vi "Main.vi"(11 "Args":string[](array[string])) -> (2 "Output":string, 3 "Return Status":i32)   [LabVIEW 2019, in "MicronTemplateService.lvlib"]
uses:
  MicronTemplateService.lvlib
  vi.lib/Micron/Base/Server/Service/ServiceBase.lvclass
  vi.lib/Micron/Base/Server/Service/Typedefs/MicronArgs.ctl
  Core/MicronTemplateCore.lvclass
  <vilib>/Utility/error.llb/DialogType.ctl
  <vilib>/SLL Toolkit/SLL Queued State Machine/Queue Driver/Create Queue.vi
  <vilib>/SLL Toolkit/SLL Queued State Machine/Queue Driver/Enqueue an Item to Queue.vi
  <vilib>/SLL Toolkit/SLL Queued State Machine/Queue Driver/Dequeue Queue.vi
  <vilib>/SLL Toolkit/SLL Queued State Machine/Queue Driver/Enstack an Item to Queue.vi
  Core/Methods/Add.vi
  <vilib>/SLL Toolkit/SLL Queued State Machine/Queue Driver/Enqueue N Items.vi
  <vilib>/SLL Toolkit/SLL Queued State Machine/Queue Driver/Flush Queue.vi
  <vilib>/SLL Toolkit/SLL Queued State Machine/Queue Driver/Release Queue.vi
  vi.lib/Micron/Base/Server/Message/MessageBase.lvclass
  <vilib>/SLL Toolkit/SLL Queued State Machine/SLL QSM.lvlib
  vi.lib/Micron/gRPC/Server/Service/GRPCService.lvclass
  <vilib>/SLL Toolkit/SLL String/SLL String.lvlib
panel:
  in  "Mode":enum32{"Service", "Manual"}(tab)
  in  "Connection String":string="localhost:50051"
  out "Network":string
  out "ServiceID":string
  out "Last Command":string
  out "Payload":string
  out "Last Message Timestamp":string
  in  "Command":string(combo)
  in  "Run":bool
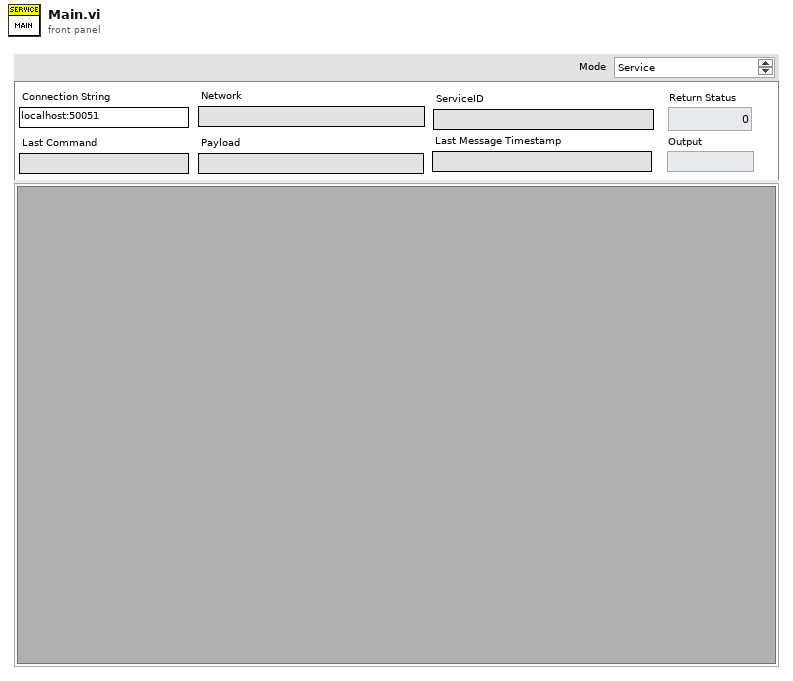
[diagram p1: front panel]
types:
  T1 = typedef "MicronServer.lvlib/ServiceBase.lvclass/MicronArgs.ctl" = cluster{"Connection":string, "Network":string, "ServiceID":string, "Port":i32, "FullyQualifiedName":string, "UI":string, "Args":string[]}
  T2 = cluster{"Flags":cluster{"Source Code?":bool}, "MicronServer":refnum<class "ServiceBase.lvclass">, "Service":T1, "UI":cluster{"Hide?":bool, "SubPanel":refnum<vi>}, "CommandMap":map{string, path}, "ManualCommandVI":refnum<vi>}
  T3 = enum32{"Invalid", "Standard", "Closed", "Hidden", "Minimized", "Maximized"}
  T4 = enum8{"Enabled", "Disabled", "Disabled and Grayed Out"}
  T5 = typedef "DialogType.ctl" = u16
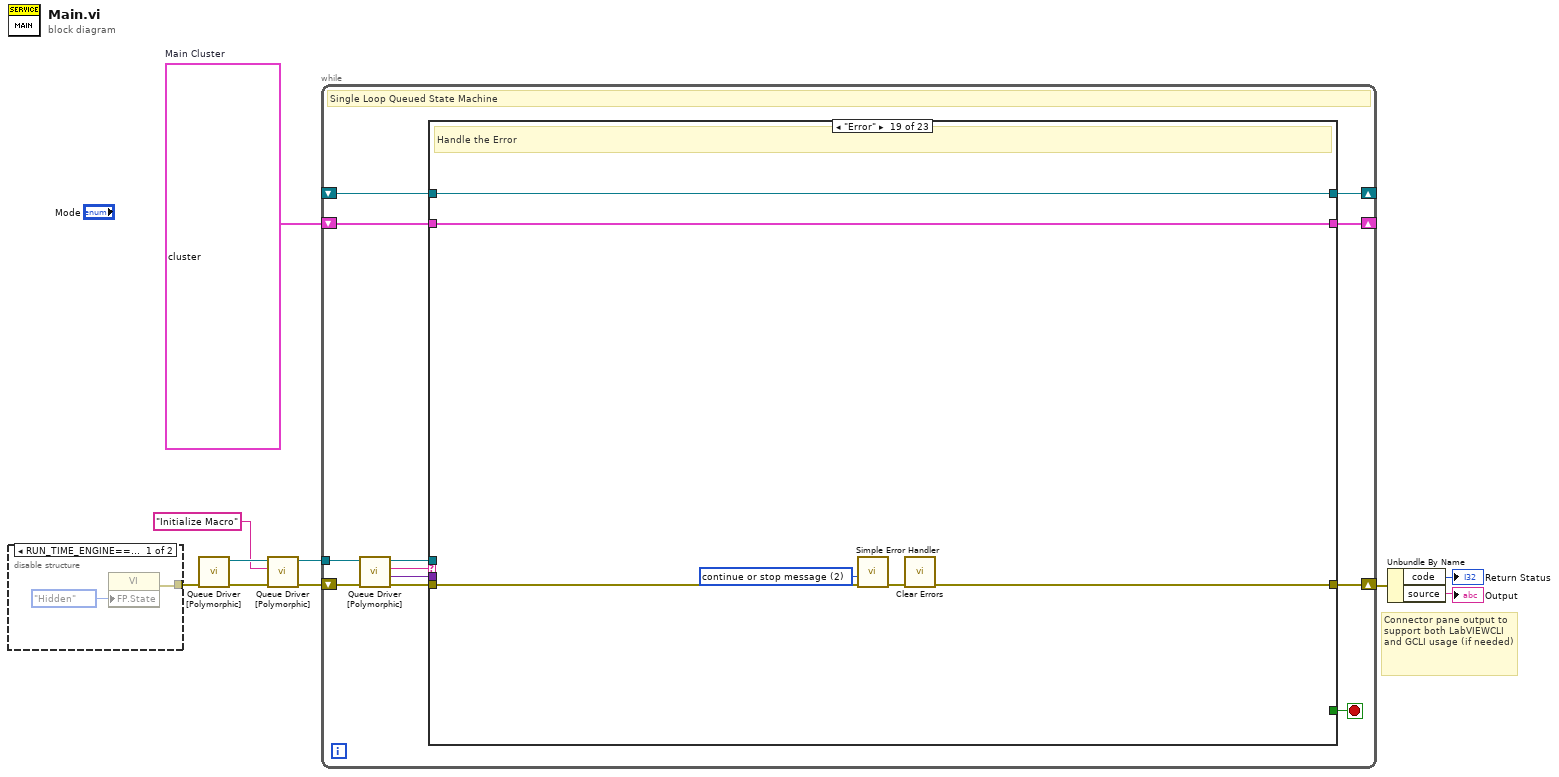
[diagram p0: block diagram]
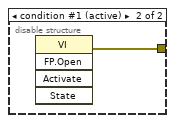
[diagram p2: hidden frame]
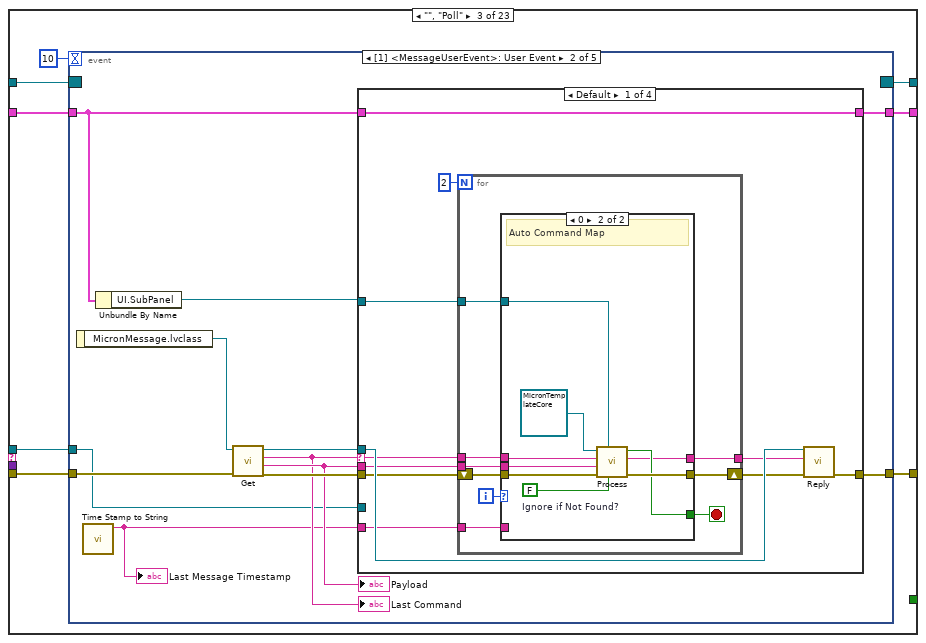
[diagram p5: hidden frame]
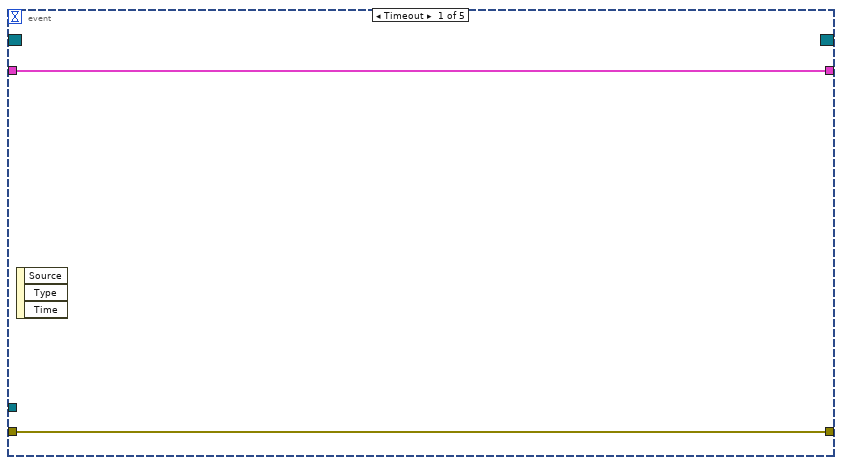
[diagram p6: hidden frame]
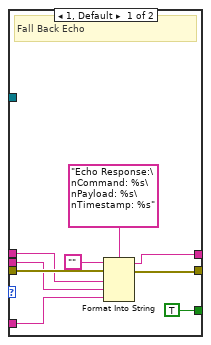
[diagram p7: hidden frame]
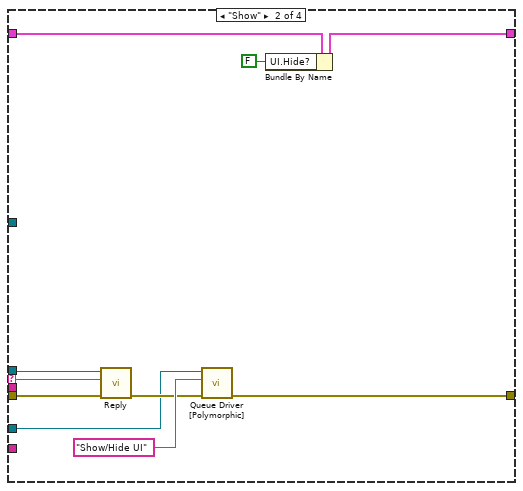
[diagram p8: hidden frame]
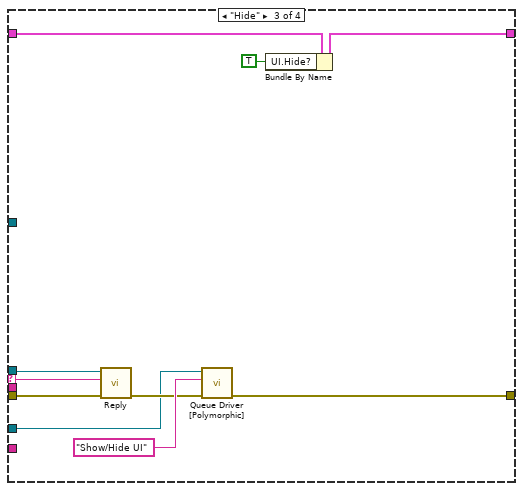
[diagram p9: hidden frame]
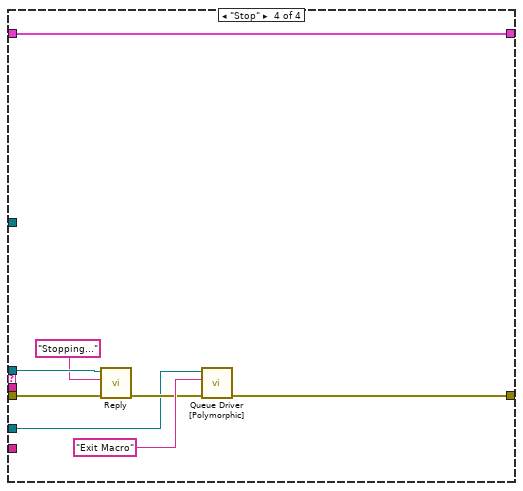
[diagram p10: hidden frame]
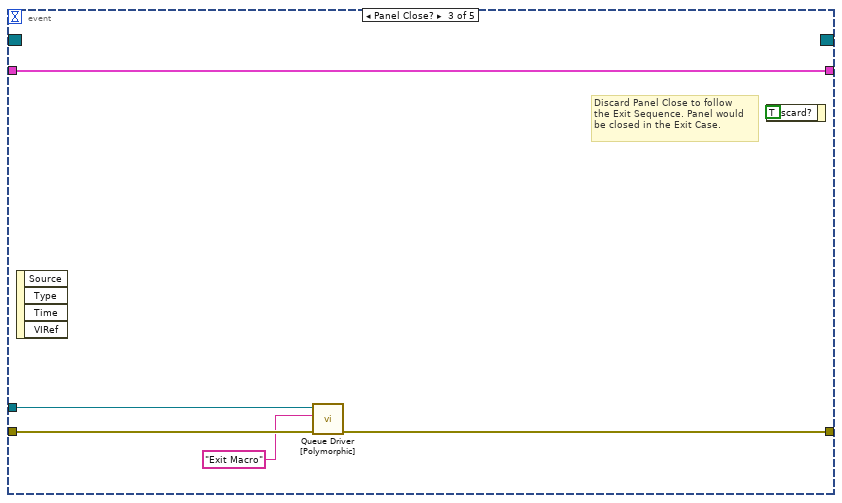
[diagram p11: hidden frame]
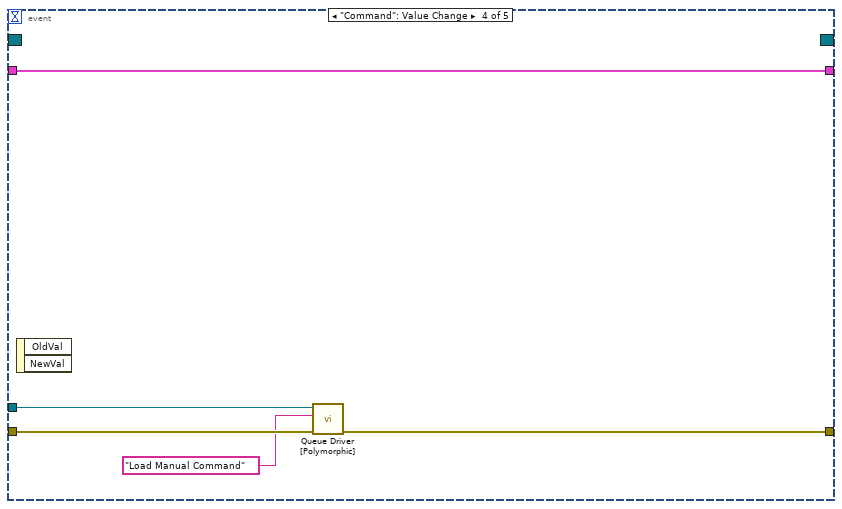
[diagram p12: hidden frame]
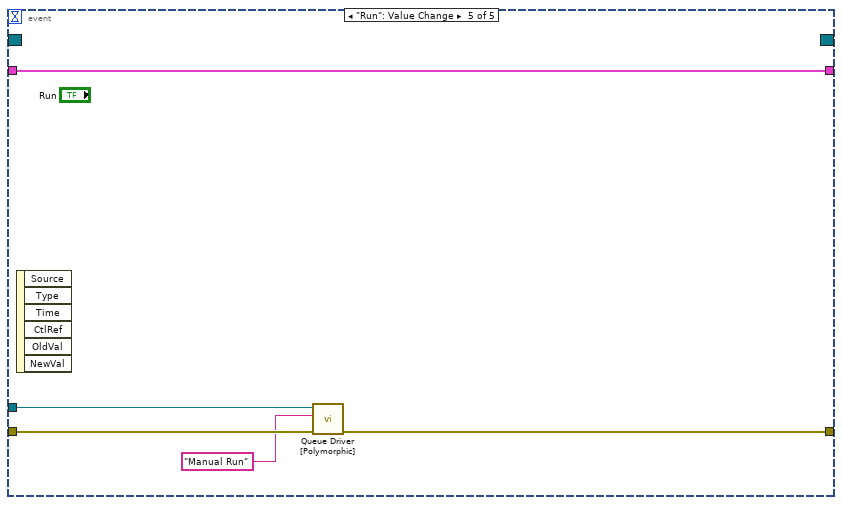
[diagram p13: hidden frame]
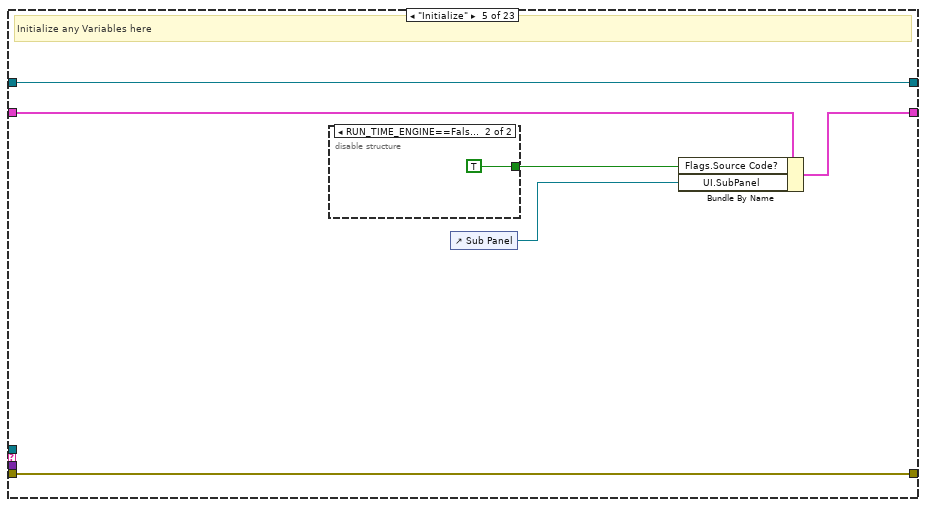
[diagram p15: hidden frame]
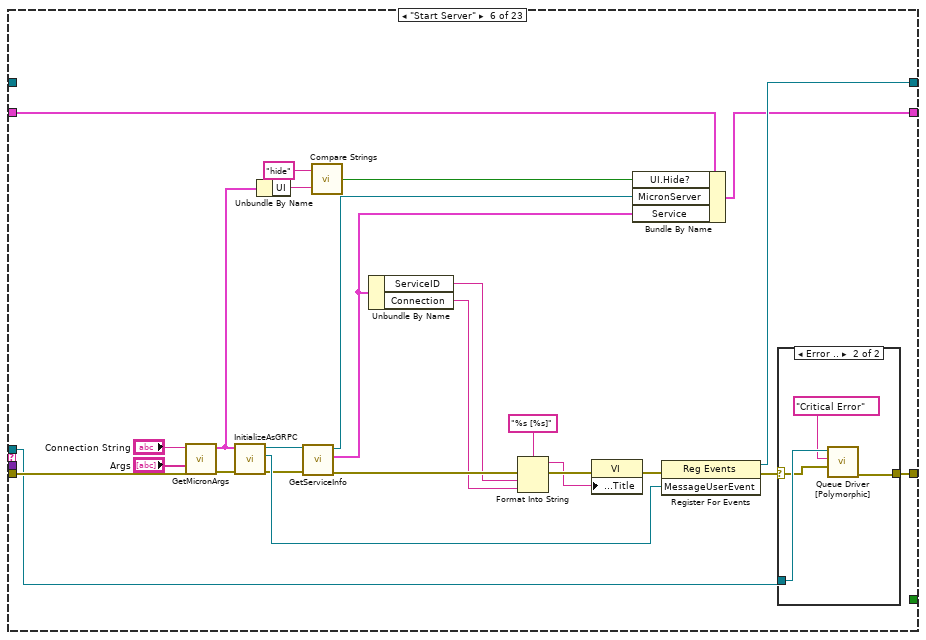
[diagram p17: hidden frame]
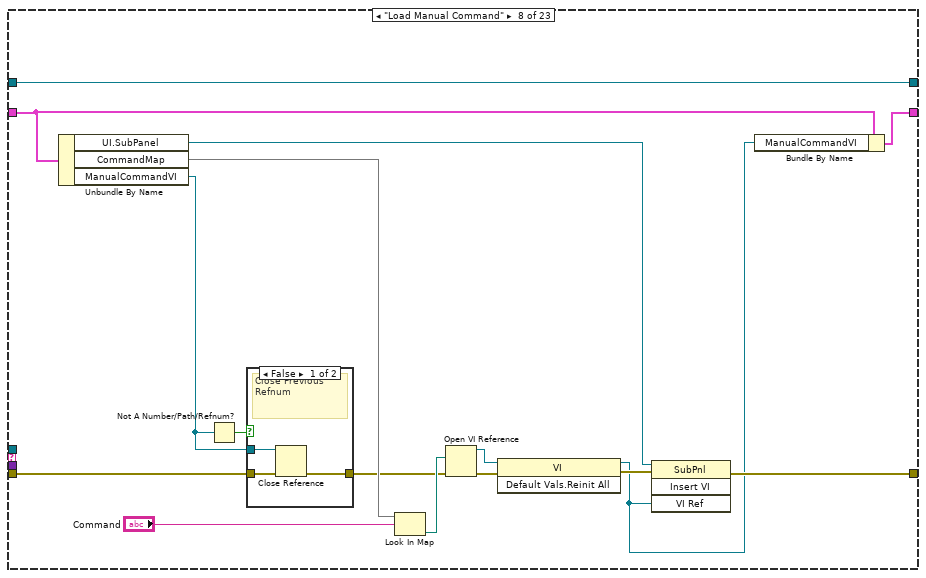
[diagram p20: hidden frame]
diagram:
  w7 = T2 {"Flags"={"Source Code?"=FALSE}, "MicronServer"=refnum, "Service"={"Connection"="", "Network"="", "ServiceID"="", "Port"=0, "FullyQualifiedName"="", "UI"="", "Args"=[]}, "UI"={"Hide?"=FALSE, "SubPanel"=refnum}, "CommandMap"={}, "ManualCommandVI"=refnum}  # Main Cluster
  # "Connector pane output to support both LabVIEWCLI and GCLI usage (if needed)"
  n1 = disable-structure shown="RUN_TIME_ENGINE==True, Default" {
    disable-tunnel: [w11 w13] -> w1
    frame condition #0 {
      n2 = property class="VI"("FP.State"=T3."Hidden" ("Front Panel Window:State")) -> (error out=w11:errorcluster)  [unwired: 2 in, 1 out]
    }
    frame condition #1 (active) {
      n3 = invoke class="VI" method="FP.Open"() -> (error out=w13:errorcluster)  [unwired: 5 in, 4 out]
    }
  }
  n4 = call-poly <vilib>:"Queue Driver [Polymorphic].vi"("Error In"=w1) -> ("Error Out"=w5:errorcluster, "Queue Ref"=w9:refnum<queue>)  [unwired: 9 in]
  n5 = call-poly <vilib>:"Queue Driver [Polymorphic].vi"("Error In"=w5, "Item to Add"="Initialize Macro", "Queue Ref In"=w9) -> ("Error Out"=w6:errorcluster, "Queue Ref Out"=w10:refnum<queue>)  [unwired: 7 in]
  n6 = while "SLL Queued State Machine" {
    shift-right: [w23] -> w4
    shift-left: w6 -> [w25]
    shift-right: [w21] -> _
    shift-left: _ -> [w20]
    shift-right: [w19] -> _
    shift-left: w7 -> [w18]
    tunnel: w10 -> [w16]
    stop <- w22 stop-if-true
    # "Single Loop Queued State Machine"
    n7 = call-poly <vilib>:"Queue Driver [Polymorphic].vi"("Error In"=w25, "Queue Ref In"=w16) -> ("Error Out"=w24:errorcluster, "Data"=w14:variant, "Dequeue"=w17:string, "Queue Ref Out"=w15:refnum<queue>)  [unwired: 6 in]
    n8 = case "QSM Case Structure" shown="\"Error\"" w17 {
      selector: w17 -> [_ _ _ _ _ _ _ _ _ _ _ _ _ _ _ _ _ w283 _ _ _ _ _]
      tunnel: w24 -> [w28 w31 w37 w138 w140 w169 w179 w195 w206 w212 w230 w244 w252 w265 w269 w277 w282 w286 w298 w303 w323 w328 w351]
      tunnel: [w28 w31 w38 w138 w140 w147 w179 w190 w202 w212 w224 w244 w251 w265 w268 w276 w282 w289 w296 w309 w323 w324 w348] -> w23
      tunnel: [_ _ _ _ _ _ _ _ _ _ _ _ _ _ _ _ _ _ _ _ _ _ TRUE] -> w22
      tunnel: [w27 w30 w36 w137 w144 w171 w178 w194 w209 w211 w235 w249 w254 w264 w271 w279 w281 w292 w295 w311 w322 w331 w336] -> w21
      tunnel: w20 -> [w27 w30 w35 w137 w144 _ w178 w194 w209 w211 w235 w249 w254 w264 w271 w279 w281 w292 w295 w311 w322 w331 w336]
      tunnel: [w26 w29 w33 w136 w141 w167 w177 w187 w208 w210 w221 w246 w253 w263 w270 w273 w280 w291 w294 w310 w321 w330 w350] -> w19
      tunnel: w18 -> [w26 w29 w34 w136 w142 w170 w177 w188 w208 w210 w222 w246 w253 w263 w270 w278 w280 w291 w294 w310 w321 w330 w350]
      tunnel: w15 -> [_ _ w32 _ _ w146 _ _ _ _ _ _ _ _ w267 w274 _ _ _ w299 _ _ w341]
      tunnel: w14 -> [_ _ _ _ _ _ _ _ _ _ _ _ _ _ _ _ _ _ _ w304 _ _ _]
      frame "/--------------- Read Me -----------------/" {
        # "General Purpose Queue Based State Machine for Any Use Case (main application, module, pop up message etc)\n\nAdvantages:\n1. Lean Project Code Base (dependencies are in vilib).\n2. This template can be safely used in multiple parallel running modules without any issues.\n3. This template can also be safely used even in cases where the VI is configured to be a clone, where multiple \ninstances of the VI could be executing concurrently.\n\nHow to Use:\n1. Add necessary items to the Main Cluster.\n2. Use the Polymorphic Queue Driver for doing any queue operations. \n3. Use \"Macros\" section for defining any list of state calls, which could be used in multiple places. \nEx: Initialize Macro, might be needed if we need to any reinitialization."
      }
      frame "/------------------ Poll -------------------/" {
      }
      frame "", "Poll" {
        n9 = event shown="[1] <MessageUserEvent>: User Event" {
          selector: w35 -> [_ _ _ _ _]
          dyn-events: [_ _ _ _ _] -> w36
          timeout: 10 -> [_ _ _ _ _]
          tunnel: [w41 w50 w124 w129 w134] -> w38
          tunnel: w37 -> [w41 w51 w125 w130 w135]
          tunnel: w34 -> [w40 w43 w123 w128 w133]
          tunnel: [w40 w45 w123 w128 w133] -> w33
          tunnel: w32 -> [_ w46 w121 w127 w132]
          event Timeout {
            n10 = event-data() -> ()  [unwired: 1 in, 3 out]
          }
          event User Event {
            n11 = event-data() -> ("MicronMessage.lvclass"=w49:refnum<class "MessageBase.lvclass">)  [unwired: 1 in]
            n12 = call <vilib>:"Time Stamp to String.vi"() -> ("Output String"=w44:string)  [unwired: 11 in]
            "Last Message Timestamp" <- w44
            n13 = Unbundle By Name(w43) -> ("UI.SubPanel"=w42:refnum<vi>)
            n14 = call-dynamic "Get.vi"("error in (no error)"=w51, "MicronMessage in"=w49) -> ("error out"=w53:errorcluster, "Payload"=w48:string, "Command"=w47:string, "MicronMessage out"=w52:refnum<class "MessageBase.lvclass">)  [unwired: 6 in]
            "Payload" <- w48
            "Last Command" <- w47
            n15 = case shown="Default" w47 {
              selector: w47 -> [w61 w95 w105 _]
              tunnel: w53 -> [w59 w101 w111 w119]
              tunnel: w52 -> [w64 w100 w110 w118]
              tunnel: [w63 w97 w107 w114] -> w50
              tunnel: w48 -> [w60 _ _ _]
              tunnel: w46 -> [_ w96 w106 w113]
              tunnel: w43 -> [w62 w94 w104 w112]
              tunnel: [w62 w93 w103 w112] -> w45
              tunnel: w44 -> [w55 _ _ _]
              tunnel: w42 -> [w57 _ _ _]
              frame Default {
                n16 = for {
                  N: 2 -> [_]
                  tunnel: w61 -> [w73]
                  tunnel: w60 -> [w72]
                  tunnel: w57 -> [w69]
                  shift-right: [w70] -> w58
                  shift-left: w59 -> [w71]
                  tunnel: w55 -> [w66]
                  tunnel: [w65] -> w54
                  i -> [w67]
                  stop <- w68 stop-if-true
                  n17 = case shown="0" w67 {
                    tunnel: w73 -> [w78 w91]
                    tunnel: w72 -> [w77 w90]
                    tunnel: w71 -> [w80 w89]
                    tunnel: [w79 w88] -> w70
                    tunnel: w69 -> [_ w87]
                    tunnel: [TRUE ("Match Present?") w85] -> w68
                    tunnel: w66 -> [w76 _]
                    tunnel: [w74 w84] -> w65
                    frame 1, Default {
                      # "Fall Back Echo"
                      n18 = Format Into String(format string="Echo Response:\nCommand: %s\nPayload: %s\nTimestamp: %s", initial string="", error in=w80, w78, w77, w76) -> (resulting string=w74:string, error out=w79:errorcluster)
                    }
                    frame 0 {
                      w83 = FALSE  # Ignore if Not Found?
                      # "Auto Command Map"
                      n19 = call "Process.vi"("Ignore if Not Found?"=w83, "SubPnl Refnum"=w87, "error in (no error)"=w89, "Payload"=w90, "Command"=w91, "Core Class"=refnum<class "MicronTemplateCore.lvclass"> refnum ("MicronTemplateCore.lvclass")) -> ("error out"=w88:errorcluster, "Response"=w84:string, "Match Present?"=w85:bool)  [unwired: 3 in]
                    }
                  }
                }
                n20 = call-dynamic "Reply.vi"("error in (no error)"=w58, "Response"=w54, "MicronMessage in"=w64) -> ("error out"=w63:errorcluster)  [unwired: 7 in, 1 out]
              }
              frame "Show" {
                n21 = call-dynamic "Reply.vi"("error in (no error)"=w101, "Response"=w95, "MicronMessage in"=w100) -> ("error out"=w98:errorcluster)  [unwired: 7 in, 1 out]
                n22 = call-poly <vilib>:"Queue Driver [Polymorphic].vi"("Error In"=w98, "Item to Add"="Show/Hide UI" ("Enqueue"), "Queue Ref In"=w96) -> ("Error Out"=w97:errorcluster)  [unwired: 7 in, 1 out]
                n23 = Bundle By Name(cluster=w94, "UI.Hide?"=FALSE) -> (w93:T2)
              }
              frame "Hide" {
                n24 = call-dynamic "Reply.vi"("error in (no error)"=w111, "Response"=w105, "MicronMessage in"=w110) -> ("error out"=w108:errorcluster)  [unwired: 7 in, 1 out]
                n25 = call-poly <vilib>:"Queue Driver [Polymorphic].vi"("Error In"=w108, "Item to Add"="Show/Hide UI" ("Enqueue"), "Queue Ref In"=w106) -> ("Error Out"=w107:errorcluster)  [unwired: 7 in, 1 out]
                n26 = Bundle By Name(cluster=w104, "UI.Hide?"=TRUE) -> (w103:T2)
              }
              frame "Stop" {
                n27 = call-dynamic "Reply.vi"("error in (no error)"=w119, "Response"="Stopping...", "MicronMessage in"=w118) -> ("error out"=w115:errorcluster)  [unwired: 7 in, 1 out]
                n28 = call-poly <vilib>:"Queue Driver [Polymorphic].vi"("Error In"=w115, "Item to Add"="Exit Macro" ("Enqueue"), "Queue Ref In"=w113) -> ("Error Out"=w114:errorcluster)  [unwired: 7 in, 1 out]
              }
            }
          }
          event Panel Close? {
            # "Discard Panel Close to follow\nthe Exit Sequence. Panel would\nbe closed in the Exit Case."
            n29 = event-data() -> ()  [unwired: 1 in, 4 out]
            n30 = call-poly <vilib>:"Queue Driver [Polymorphic].vi"("Error In"=w125, "Item to Add"="Exit Macro" ("Enqueue"), "Queue Ref In"=w121) -> ("Error Out"=w124:errorcluster)  [unwired: 7 in, 1 out]
            n31 = event-data("Discard?"=TRUE) -> ()  [unwired: 1 in, 1 out]
          }
          event "Command": Value Change {
            n32 = event-data() -> ()  [unwired: 1 in, 2 out]
            n33 = call-poly <vilib>:"Queue Driver [Polymorphic].vi"("Error In"=w130, "Item to Add"="Load Manual Command" ("Enqueue"), "Queue Ref In"=w127) -> ("Error Out"=w129:errorcluster)  [unwired: 7 in, 1 out]
          }
          event "Run": Value Change {
            n34 = event-data() -> ()  [unwired: 1 in, 6 out]
            n35 = call-poly <vilib>:"Queue Driver [Polymorphic].vi"("Error In"=w135, "Item to Add"="Manual Run" ("Enqueue"), "Queue Ref In"=w132) -> ("Error Out"=w134:errorcluster)  [unwired: 7 in, 1 out]
          }
        }
      }
      frame "/--------------- Initialize -----------------/" {
      }
      frame "Initialize" {
        # "Initialize any Variables here"
        n36 = disable-structure shown="RUN_TIME_ENGINE==False" {
          disable-tunnel: [_ TRUE] -> w143
          frame condition #0 {
          }
          frame condition #1 (active) {
          }
        }
        n37 = control-ref of="Sub Panel"() -> (w139:refnum<vi>)
        n38 = Bundle By Name(cluster=w142, "Flags.Source Code?"=w143, "UI.SubPanel"=w139) -> (w141:T2)
      }
      frame "Start Server" {
        n39 = call "GetMicronArgs.vi"("error in (no error)"=w169, "Args"="Args", "Default Connection String"="Connection String") -> ("error out"=w164:errorcluster, "Micron Args"=w161:T1)  [unwired: 7 in]
        n40 = call "InitializeAsGRPC.vi"("error in (no error)"=w164, "Service"=w161) -> ("error out"=w165:errorcluster, "MessageUserEvent"=w168:refnum<user-event>, "MicronServer"=w163:refnum<class "ServiceBase.lvclass">)  [unwired: 7 in]
        n41 = Unbundle By Name(w161) -> ("UI"=w160:string)
        n42 = call-dynamic "GetServiceInfo.vi"("error in (no error)"=w165, "ServiceBase in"=w163) -> ("error out"=w156:errorcluster, "Service"=w154:T1, "ServiceBase out"=w162:refnum<class "ServiceBase.lvclass">)  [unwired: 7 in]
        n43 = call <vilib>:"Compare Strings.vi"("y"=w160, "x"="hide") -> ("Equal?"=w158:bool)
        n44 = Unbundle By Name(w154) -> ("ServiceID"=w151:string, "Connection"=w150:string)
        n45 = Format Into String(format string="%s [%s]", error in=w156, w151, w150) -> (resulting string=w149:string, error out=w153:errorcluster)  [unwired: 1 in]
        n46 = property class="VI"(error in=w153, "Front Panel.Title"=w149) -> (error out=w155:errorcluster)  [unwired: 1 in, 1 out]
        n47 = Bundle By Name(cluster=w170, "UI.Hide?"=w158, "MicronServer"=w162, "Service"=w154) -> (w167:T2)
        n48 = register-events(error in=w155, w168) -> (reference out=w171:refnum<event-registration>, error out=w148:errorcluster)  [unwired: 1 in]
        n49 = case shown="Error .." w148 {
          selector: w148 -> [w172 w174]
          tunnel: [w172 w173] -> w147
          tunnel: w146 -> [_ w176]
          frame No Error {
          }
          frame Error {
            n50 = call-poly <vilib>:"Queue Driver [Polymorphic].vi"("Data (Optional)"=w174, "Item to Add"="Critical Error", "Queue Ref In"=w176) -> ("Error Out"=w173:errorcluster)  [unwired: 7 in, 1 out]
          }
        }
      }
      frame "/---------- Custom Case Splitter ----------/" {
      }
      frame "Load Manual Command" {
        n51 = Unbundle By Name(w188) -> ("UI.SubPanel"=w189:refnum<vi>, "CommandMap"=w193:map{string, path}, "ManualCommandVI"=w184:refnum<vi>)
        n52 = Not A Number/Path/Refnum?(number/path/refnum=w184) -> (NaN/Path/Refnum?=w185:bool)
        n53 = case shown="False" w185 {
          tunnel: w195 -> [w198 w199]
          tunnel: [w197 w199] -> w186
          tunnel: w184 -> [w196 _]
          frame False {
            # "Close Previous Refnum"
            n54 = Close Reference(reference=w196, error in (no error)=w198) -> (error out=w197:errorcluster)
          }
          frame True {
          }
        }
        n55 = Look In Map(map=w193, key="Command") -> (value=w191:path)  [unwired: 1 in, 1 out]
        n56 = Open VI Reference(vi path=w191, error in (no error)=w186) -> (vi reference=w183:refnum<vi>, error out=w182:errorcluster)  [unwired: 4 in]
        n57 = invoke class="VI" method="Default Vals.Reinit All"(reference=w183, error in=w182) -> (reference out=w180:refnum<vi>, error out=w181:errorcluster)  [unwired: 1 in, 1 out]
        n58 = invoke class="SubPnl" method="Insert VI"(reference=w189, error in=w181, "VI Ref"=w180) -> (error out=w190:errorcluster)  [unwired: 1 in, 3 out]
        n59 = Bundle By Name(cluster=w188, "ManualCommandVI"=w180) -> (w187:T2)
      }
      frame "Manual Run" {
        n60 = Unbundle By Name(w208) -> ("ManualCommandVI"=w207:refnum<vi>)
        n61 = property on="Run" class="Bool"(error in=w206, "DisabledEnum"=T4."Disabled and Grayed Out" ("Disabled")) -> (error out=w204:errorcluster)  [unwired: 1 in, 1 out]
        n62 = invoke class="VI" method="Run VI"(reference=w207, error in=w204, "Wait until done"=TRUE ("Wait Until Done")) -> (error out=w203:errorcluster)  [unwired: 2 in, 4 out]
        n63 = property on="Run" class="Bool"(error in=w203, "DisabledEnum"=T4."Enabled" ("Disabled")) -> (error out=w202:errorcluster)  [unwired: 1 in, 1 out]
      }
      frame "/-------------- User Interface --------------/" {
        # "Duplicate this case to create additional case splitters for readability"
      }
      frame "Populate Commands" {
        w226 = map{string, path} {}  # Size: 0
        n64 = vi-ref "MicronTemplateCore.lvclass:Add.vi"() -> (w231:refnum<vi>)
        n65 = property class="VI"(reference=w231, error in=w230) -> (reference out=w214:refnum<vi>, error out=w229:errorcluster, "Library"=w234:refnum<vi>)
        n66 = invoke class="Library" method="Get All Descendents"(reference=w234, error in=w229, "Type"="VI", "Exclude Dependencies"=TRUE ("ExcludeDependencies")) -> (reference out=w216:refnum<vi>, error out=w227:errorcluster, "All Descendents"=w228:refnum<vi>[])  [unwired: 3 in, 4 out]
        n67 = for {
          tunnel: w228 -> [w243] mode=indexing
          shift-right: [w241] -> w225
          shift-left: w227 -> [w242]
          shift-right: [w238] -> w220
          shift-left: w226 -> [w239]
          tunnel: [w237] -> w223 mode=indexing
          tunnel: [w236] -> w218 mode=indexing
          n68 = property class="ProjectItem"(reference=w243, error in=w242) -> (reference out=w236:refnum<vi>, error out=w241:errorcluster, "Name"=w237:string, "Path"=w240:path)
          n69 = Insert Into Map(map in=w239, key=w237, value=w240) -> (map out=w238:map{string, path})  [unwired: 2 out]
        }
        n70 = Close Reference(reference=w218, error in (no error)=w225) -> (error out=w219:errorcluster)
        n71 = Bundle By Name(cluster=w222, "CommandMap"=w220) -> (w221:T2)
        n72 = Close Reference(reference=w216, error in (no error)=w219) -> (error out=w217:errorcluster)
        n73 = Close Reference(reference=w214, error in (no error)=w217) -> (error out=w215:errorcluster)
        n74 = property on="Command" class="CmbBox"(error in=w215, "Strings[]"=w223, "Value"="") -> (error out=w224:errorcluster)  [unwired: 1 in, 1 out]
      }
      frame "Update UI" {
        # "Update Front Panel Controls in this Case"
        n75 = Unbundle By Name(w246) -> ("Service.Network"=→"Network":string, "Service.ServiceID"=→"ServiceID":string, "Service.Connection"=w245:string)
        n76 = local write "Connection String"(w245) -> ()
      }
      frame "Show/Hide UI" {
        # "Update Front Panel Controls in this Case"
        n77 = Unbundle By Name(w253) -> ("UI.Hide?"=w250:bool)
        n78 = case "Hide?" shown="True" w250 {
          tunnel: w252 -> [w256 w260]
          tunnel: [w255 w259] -> w251
          frame True {
            n79 = property class="VI"(error in=w256, "FP.State"=T3."Hidden" ("Front Panel Window:State"), "FP:Transparency"=u8 100 ("Front Panel Window:Transparency")) -> (error out=w255:errorcluster)  [unwired: 1 in, 1 out]
          }
          frame False {
            n80 = property class="VI"(error in=w260, "FP.State"=T3."Standard" ("Front Panel Window:State"), "FP:Transparency"=u8 0 ("Front Panel Window:Transparency")) -> (error out=w259:errorcluster)  [unwired: 1 in, 1 out]
          }
        }
      }
      frame "/----------------- Macros -----------------/" {
      }
      frame "Initialize Macro" {
        w266 = string[] ["Initialize", "Start Server", "Show/Hide UI", "Populate Commands", "Update UI"]  # Initialize Macro
        n81 = call-poly <vilib>:"Queue Driver [Polymorphic].vi"("Error In"=w269, "Enqueue N"=w266, "Queue Ref In"=w267) -> ("Error Out"=w268:errorcluster)  [unwired: 7 in, 1 out]
      }
      frame "Exit Macro" {
        n82 = call-poly <vilib>:"Queue Driver [Polymorphic].vi"("Error In"=w277, "Enqueue N"=string[] ["Show/Hide UI", "Close References", "Exit"], "Queue Ref In"=w274) -> ("Error Out"=w276:errorcluster)  [unwired: 7 in, 1 out]
        n83 = Bundle By Name(cluster=w278, "UI.Hide?"=TRUE) -> (w273:T2)
      }
      frame "/-------------- Error Handler--------------/" {
      }
      frame Default {
        # "Undefined Case/Spelling Errors - Show Message to Developer"
        n84 = property class="VI"(error in=w286) -> (error out=w285:errorcluster, "Name"=w284:string)  [unwired: 1 in, 1 out]
        n85 = Format Into String(format string="\"%s\" in the VI - %s" ("message"), initial string="Undefined case - ", error in=w285, w283, w284) -> (resulting string=w287:string, error out=w289:errorcluster)
        n86 = One Button Dialog(message=w287) -> ()  [unwired: 1 in, 1 out]
      }
      frame "Error" {
        w293 = T5 2 items=["no dialog", "OK message", "continue or stop message", "OK message + warnings", "continue/stop + warnings"] ("type of dialog (OK msg:1)")
        # "Handle the Error"
        n87 = call <vilib>:"Simple Error Handler.vi"("type of dialog (OK msg:1)"=w293, "error in (no error)"=w298) -> ("error out"=w297:errorcluster)  [unwired: 3 in, 4 out]
        n88 = call <vilib>:"Clear Errors.vi"("error in (no error)"=w297) -> ("error out"=w296:errorcluster)  [unwired: 5 in, 1 out]
      }
      frame "Critical Error" {
        n89 = Unbundle By Name(w310) -> ("Flags.Source Code?"=w306:bool, "UI.Hide?"=w308:bool)
        n90 = Variant To Data(error in=w303, type=w303, Variant=w304) -> (data=w301:errorcluster, error out=w302:errorcluster)
        n91 = Merge Errors(w302, w301) -> (w300:errorcluster)
        n92 = Not(x=w308) -> (.not. x?=w307:bool)
        n93 = Or(x=w306, y=w307) -> (x .or. y?=w305:bool)
        n94 = case "Show Error Pop Up?" shown="True" w305 {
          tunnel: w300 -> [w316 w319]
          tunnel: [w314 w317] -> w309
          tunnel: w299 -> [w313 _]
          frame False {
            # "#TBD Log Error"
            # "Stop Service"
            n95 = call <vilib>:"Clear Errors.vi"("error in (no error)"=w316) -> ("error out"=w315:errorcluster)  [unwired: 5 in, 1 out]
            n96 = call-poly <vilib>:"Queue Driver [Polymorphic].vi"("Error In"=w315, "Item to Add"="Exit Macro", "Queue Ref In"=w313) -> ("Error Out"=w314:errorcluster)  [unwired: 7 in, 1 out]
          }
          frame True {
            w320 = T5 2 items=["no dialog", "OK message", "continue or stop message", "OK message + warnings", "continue/stop + warnings"] ("type of dialog (OK msg:1)")
            # "Source Code or Show UI Mode"
            n97 = call <vilib>:"Simple Error Handler.vi"("type of dialog (OK msg:1)"=w320, "error in (no error)"=w319) -> ("error out"=w318:errorcluster)  [unwired: 3 in, 4 out]
            n98 = call <vilib>:"Clear Errors.vi"("error in (no error)"=w318) -> ("error out"=w317:errorcluster)  [unwired: 5 in, 1 out]
          }
        }
      }
      frame "/------------------- Exit --------------------/" {
      }
      frame "Close References" {
        n99 = Unbundle By Name(w330) -> ("UI.SubPanel"=w325:refnum<vi>, "ManualCommandVI"=w327:refnum<vi>)
        n100 = Not A Number/Path/Refnum?(number/path/refnum=w327) -> (NaN/Path/Refnum?=w329:bool)
        n101 = case shown="False" w329 {
          tunnel: w328 -> [w334 w335]
          tunnel: [w333 w335] -> w326
          tunnel: w327 -> [w332 _]
          frame False {
            # "Close Previous Refnum"
            n102 = Close Reference(reference=w332, error in (no error)=w334) -> (error out=w333:errorcluster)
          }
          frame True {
          }
        }
        n103 = Close Reference(reference=w325, error in (no error)=w326) -> (error out=w324:errorcluster)
      }
      frame "Exit" {
        n104 = call-poly <vilib>:"Queue Driver [Polymorphic].vi"("Error In"=w351, "Queue Ref In"=w341) -> ("Error Out"=w352:errorcluster, "Queue Ref Out"=w340:refnum<queue>)  [unwired: 7 in, 1 out]
        n105 = call-poly <vilib>:"Queue Driver [Polymorphic].vi"("Error In"=w352, "Queue Ref In"=w340) -> ("Error Out"=w349:errorcluster)  [unwired: 9 in]
        n106 = Unregister For Events(event registration refnum=w336, error in=w349) -> (error out=w337:errorcluster)
        n107 = Unbundle By Name(w350) -> ("Flags.Source Code?"=w343:bool, "MicronServer"=w338:refnum<class "ServiceBase.lvclass">)
        n108 = call-dynamic "CloseCore.vi"("error in (no error)"=w337, "MicronServer in"=w338) -> ("error out"=w339:errorcluster)  [unwired: 8 in, 1 out]
        n109 = Call Chain() -> (call chain=w347:string[])
        n110 = Array Size(array=w347) -> (size(s)=w346:i32)
        n111 = Equal?(x=w346, y=1) -> (x = y?=w344:bool)
        n112 = And(x=w343, y=w344) -> (x .and. y?=w342:bool)
        n113 = case "Skip Panel Close when in Source\nCode and is the top most caller" shown="False" w342 {
          tunnel: w339 -> [w355 w357]
          tunnel: [w356 w357] -> w348
          frame False {
            # "Close Panel"
            n114 = invoke class="VI" method="FP.Close"() -> (error out=w354:errorcluster)  [unwired: 3 in, 2 out]
            n115 = Merge Errors(w355, w354) -> (w356:errorcluster)
          }
          frame True {
            # "Do Not Close Panel"
          }
        }
      }
    }
  }
  n116 = Unbundle By Name(w4) -> ("code"=→"Return Status":i32, "source"=→"Output":string)
